vi "UI Initialize.vi"(8 "error in (no error)":errorcluster, 11 "UI ActorTop in":refnum<class "UI_Top.lvclass">) -> (0 "error out":errorcluster, 3 "UI ActorTop out":refnum<class "UI_Top.lvclass">)   [LabVIEW 2021, in "UI_Top.lvclass"]
doc: "UI: Initialize\n2015-03-18 16:27:22\n蒋松\njiangsong@outlook.com"
uses:
  UI_Top.lvclass
  UI_Top.lvclass/UI_Top.ctl
  <userlib>/John_Lib/AbstractActorTemplate/AbstractActorTemplate/UIActorTop.lvclass
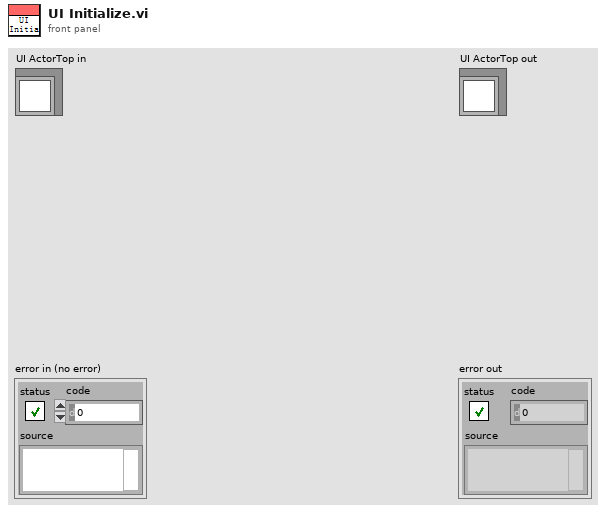
[diagram p1: front panel]
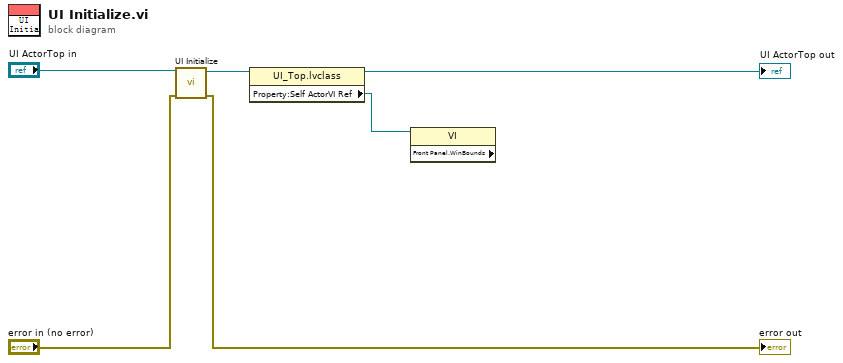
[diagram p0: block diagram]
diagram:
  n1 = call-parent "UI Initialize.vi"("error in (no error)"="error in (no error)", "UI ActorTop in"="UI ActorTop in") -> ("error out"=→"error out":errorcluster, "UI ActorTop out"=w4:refnum<class "UI_Top.lvclass">)  [unwired: 8 in]
  n2 = property class="UI_Top.lvclass"(reference=w4) -> (reference out=→"UI ActorTop out":refnum<class "UI_Top.lvclass">, "Property:Self ActorVI Ref"=w1:refnum<vi>)  [unwired: 1 in, 1 out]
  n3 = property class="VI" props=["Front Panel.WinBounds"](reference=w1) -> ()  [unwired: 1 in, 3 out]
